vi "Request Synchronous Variant.vi"(6 "Ignore Past Updates? (F)":bool, 7 "Timeout In ms (-1)":i32=-1, 8 "error in (no error)":errorcluster, 9 "Type":variant, 10 "Datum Name":string, 11 "IObserver In":refnum<class "IObserver.lvclass">) -> (0 "error out":errorcluster, 1 "timed out?":bool, 2 "Data":variant, 4 "Publication Time":timestamp)   [LabVIEW 2015, in "IObserver.lvlib" / "IObserver.lvclass"]
doc: "<License>\nCopyright © 2017 Composed Systems, LLC | All rights reserved\nwww.composed.io\n\nAuthor: Ethan Stern <ethan.stern@composed.io>\n\nThis software is provided \"AS IS\" WITHOUT WARRANTIES, either express or implied, AND IS FOR EDUCATIONAL PURPOSES ONLY.\n</License>"
uses:
  IObserver.lvclass
  IObserver.lvclass/IObserver.ctl
  SubscriptionPolicy/OneShotSubscription/OneShotSubscription.lvclass/OneShotSubscription.ctl
  Transport/QueueTransport/QueueTransport.lvclass/QueueTransport.ctl
  IMediator/SubscriptionRequest/SubscriptionRequest.lvclass/SubscriptionRequest.ctl
  AbstractMessages/PreAddressedMsg/PreAddressedMsg.lvclass/PreAddressedMsg.ctl
  IMediator/IMediator Messages/Subscribe Msg/Subscribe Msg.lvclass/Subscribe Msg.ctl
  <vilib>/ActorFramework/Message Enqueuer/Message Enqueuer.lvclass/Message Enqueuer.ctl
  <vilib>/ActorFramework/Message Enqueuer/Enqueue.vi
  AbstractMessages/PreAddressedMsg/Read Return Address.vi
  <vilib>/Utility/error.llb/Error Cluster From Error Code.vi
  <vilib>/ActorFramework/Message Priority Queue/Priority Enqueue.vi
  IMediator/SubscriptionRequest/SubscriptionRequest.lvclass
  SubscriptionPolicy/OneShotSubscription/OneShotSubscription.lvclass
  Transport/QueueTransport/QueueTransport.lvclass
  IMediator/ISubscriptionPolicy/ISubscriptionPolicy.lvclass
  IMediator/IMediator Messages/Subscribe Msg/Subscribe Msg.lvclass
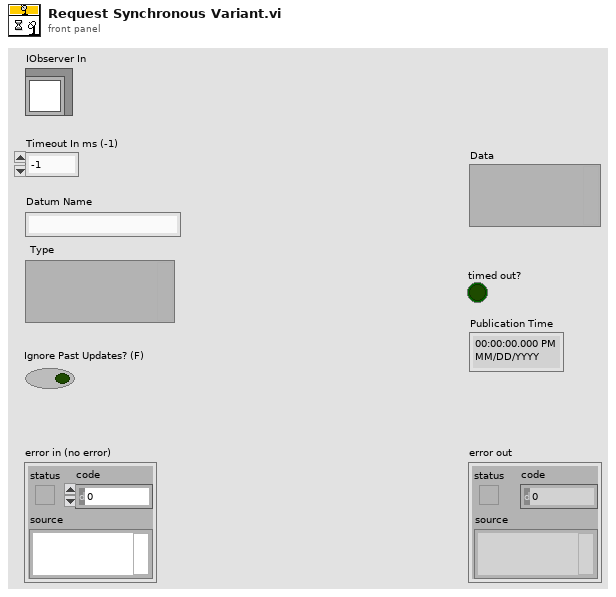
[diagram p1: front panel]
types:
  T1 = typedef "IMediator.lvlib/ISubscriptionPolicy.lvclass/ISubscriptionPolicy Reference.ctl" = refnum<data-value>
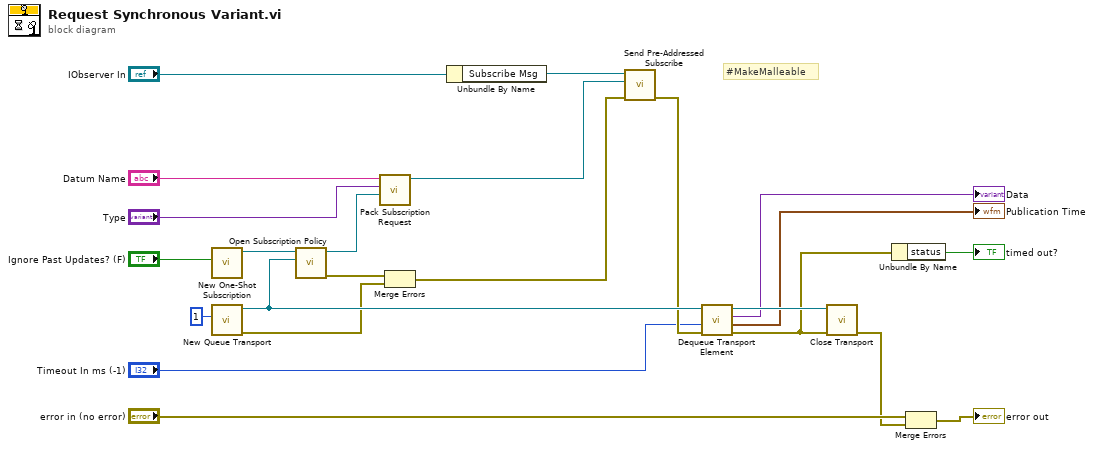
[diagram p0: block diagram]
diagram:
  # "#MakeMalleable"
  n1 = call "New One-Shot Subscription.vi"("Ignore Past Updates? (F)"="Ignore Past Updates? (F)") -> ("OneShotSubscription Out"=w18:refnum<class "OneShotSubscription.lvclass">)  [unwired: 10 in]
  n2 = call "New Queue Transport.vi"("Max Queue Size (-1)"=1 ("Max Queue Size (-1, unlimited)")) -> ("error out"=w10:errorcluster, "QueueTransport"=w12:refnum<class "QueueTransport.lvclass">)  [unwired: 9 in]
  n3 = call "Open Subscription Policy.vi"("Transport"=w12, "SubscriptionPolicy"=w18) -> ("error out"=w13:errorcluster, "Subscription Policy"=w1:T1)  [unwired: 8 in]
  n4 = call "Pack Subscription Request.vi"("Subscription Policy"=w1, "Type"="Type", "Datum Name"="Datum Name") -> ("SubscriptionRequest"=w14:refnum<class "SubscriptionRequest.lvclass">)  [unwired: 8 in]
  n5 = Merge Errors(w13, w10) -> (w11:errorcluster)
  n6 = Unbundle By Name("IObserver In") -> ("Subscribe Msg"=w15:refnum<class "Subscribe Msg.lvclass">)
  n7 = call "Send Pre-Addressed Subscribe.vi"("error in (no error)"=w11, "Subscription Request"=w14, "Subscribe Msg"=w15) -> ("error out"=w9:errorcluster)  [unwired: 8 in]
  n8 = call "Dequeue Transport Element.vi"("error in (no error)"=w9, "Timeout In ms (-1)"="Timeout In ms (-1)", "QueueTransport in"=w12) -> ("error out"=w2:errorcluster, "Publication Time"=→"Publication Time":timestamp, "Data"=→"Data":variant, "QueueTransport out"=w23:refnum<class "QueueTransport.lvclass">)  [unwired: 5 in]
  n9 = call-dynamic "Close Transport.vi"("error in (no error)"=w2, "QueueTransport in"=w23) -> ("error out"=w4:errorcluster)  [unwired: 9 in]
  n10 = Unbundle By Name(w2) -> ("status"=→"timed out?":bool)
  n11 = Merge Errors("error in (no error)", w4) -> (→"error out":errorcluster)
